vi "JSON to LVObject - Object With Member And Empty JSON Object - Returns Same Object.vi"() -> ()   [LabVIEW 2017, in "Tests.lvlib"]
uses:
  Tests.lvlib
  Weather Forecast/Weather Forecast.lvclass
  Flatten To JSON Object/Flatten To JSON Object.lvclass
  <vilib>/addons/_JKI Toolkits/Caraya/classes/Assert/Assert Equal Value and Type_Variant.vi
  <vilib>/addons/_JKI Toolkits/Caraya/classes/Test/Test.lvclass
  <vilib>/addons/_JKI Toolkits/Caraya/classes/Assert/Assert.lvclass
panel:
  out "error out":errorcluster
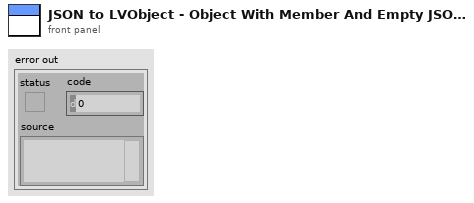
[diagram p1: front panel]
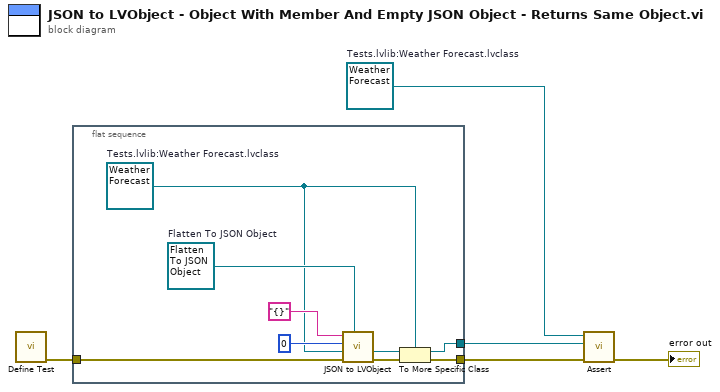
[diagram p0: block diagram]
diagram:
  w1 = refnum<class "Weather Forecast.lvclass"> refnum  # Tests.lvlib:Weather Forecast.lvclass
  n1 = call <vilib>:"Define Test.vi"() -> ("error out"=w5:errorcluster)  [unwired: 11 in]
  n2 = flat-sequence {
    tunnel: w5 -> [w13]
    tunnel: [w9] -> w4
    tunnel: [w6] -> w3
    frame #0 {
      w7 = refnum<class "Weather Forecast.lvclass"> refnum  # Tests.lvlib:Weather Forecast.lvclass
      w14 = refnum<class "Flatten To JSON Object.lvclass"> refnum  # Flatten To JSON Object
      n3 = call-dynamic "JSON to LVObject.vi"("Flatten To JSON Object in"=w14, "error in (no error)"=w13, "Object Type"=w7, "Offset"=0, "JSON"="{}") -> ("error out"=w12:errorcluster, "Object"=w8:refnum<class>)  [unwired: 5 in]
      n4 = To More Specific Class(target class=w7, reference=w8, error in=w12) -> (specific class reference=w6:refnum<class "Weather Forecast.lvclass">, error out=w9:errorcluster)
    }
  }
  n5 = call-poly <vilib>:"Assert.vi"("error in (no error)"=w4, "Y"=w3, "X"=w1) -> ("error out"=→"error out":errorcluster)  [unwired: 8 in]
